vi "UnaryClientAbortTest.vi"() -> (0 "Array of Error Description":T1)   [LabVIEW 2019]
uses:
  gRPC_ATS/TestUtility/utility.llb/array of error description.ctl
  gRPC_ATS/TestUtility/utility.llb/error description.ctl
  gRPC_ATS/TestUtility/utility.llb/error type.ctl
  Generated_client/RPC Messages/helloworld_HelloReply.ctl
  Generated_client/Generated_client.lvlib
panel:
  out "Pass":bool
  in  "error in (no error)":errorcluster
  in  "Server VI path":path=path "Generated_server/Run Service.vi"
  in  "Client VI Path":path=path "Generated_client/gRPC Client Test.vi"
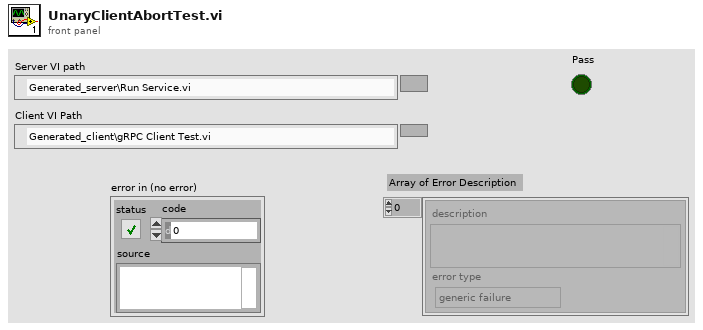
[diagram p1: front panel]
types:
  T1 = typedef "array of error description.ctl" = T2[]
  T2 = typedef "error description.ctl" = cluster{"description":string, "error type":T3}
  T3 = typedef "error type.ctl" = enum32{"generic failure", "boundary case", "precision", "expected error"}
  T4 = typedef "Generated_client.lvlib/helloworld_HelloReply.ctl" = cluster{"message":string}
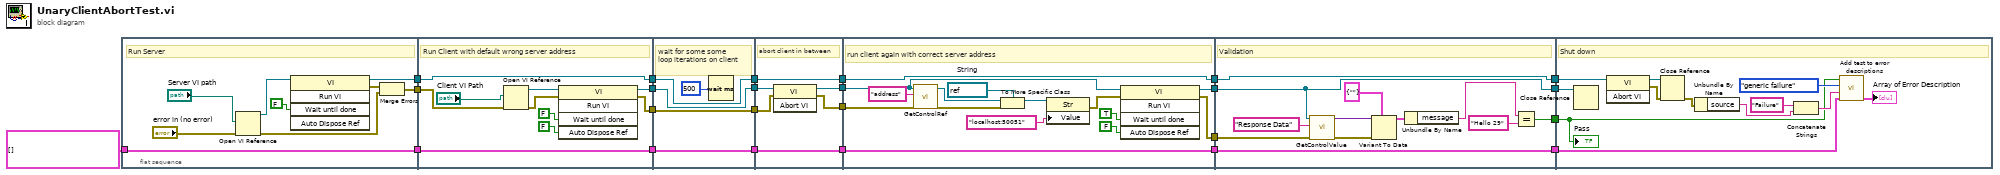
[diagram p0: block diagram]
diagram:
  n1 = flat-sequence {
    tunnel: T1 [] ("error descriptions in") -> [w29]
    tunnel: [w29] -> w23
    tunnel: [w28] -> w21
    tunnel: [w25] -> w20
    tunnel: w23 -> [w42]
    tunnel: [w42] -> w19
    tunnel: [w41] -> w17
    tunnel: w21 -> [w41]
    tunnel: w20 -> [w40]
    tunnel: [w35] -> w15
    tunnel: [w34] -> w13
    tunnel: w19 -> [w48]
    tunnel: [w48] -> w18
    tunnel: w17 -> [w47]
    tunnel: [w47] -> w16
    tunnel: w15 -> [w46]
    tunnel: [w46] -> w14
    tunnel: w13 -> [w45]
    tunnel: [w45] -> w12
    tunnel: w18 -> [w54]
    tunnel: [w54] -> w11
    tunnel: w16 -> [w53]
    tunnel: [w53] -> w9
    tunnel: w14 -> [w52]
    tunnel: [w49] -> w7
    tunnel: w12 -> [w51]
    tunnel: [w50] -> w5
    tunnel: w11 -> [w69]
    tunnel: [w69] -> w10
    tunnel: w9 -> [w68]
    tunnel: [w68] -> w8
    tunnel: w7 -> [w63]
    tunnel: [w67] -> w6
    tunnel: w5 -> [w62]
    tunnel: [w66] -> w4
    tunnel: w10 -> [w81]
    tunnel: [w81] -> w22
    tunnel: w8 -> [w80]
    tunnel: w6 -> [w77]
    tunnel: w4 -> [w75]
    tunnel: [w80] -> w3
    tunnel: [w77] -> w2
    tunnel: [w70] -> w1
    tunnel: w22 -> [w88]
    tunnel: w3 -> [w84]
    tunnel: w2 -> [w83]
    tunnel: w1 -> [w82]
    frame #0 {
      # "Run Server"
      n2 = Open VI Reference(vi path="Server VI path", error in (no error)="error in (no error)") -> (vi reference=w31:refnum<vi>, error out=w27:errorcluster)  [unwired: 4 in]
      n3 = invoke class="VI" method="Run VI"(reference=w31, "Wait until done"=FALSE ("Wait Until Done")) -> (reference out=w28:refnum<vi>, error out=w26:errorcluster)  [unwired: 3 in, 3 out]
      n4 = Merge Errors(w26, w27) -> (w25:errorcluster)
    }
    frame #1 {
      # "Run Client with default wrong server address"
      n5 = Open VI Reference(vi path="Client VI Path", error in (no error)=w40) -> (vi reference=w39:refnum<vi>, error out=w38:errorcluster)  [unwired: 4 in]
      n6 = invoke class="VI" method="Run VI"(reference=w39, error in=w38, "Wait until done"=FALSE ("Wait Until Done"), "Auto Dispose Ref"=FALSE ("Auto Dispose Reference")) -> (reference out=w35:refnum<vi>, error out=w34:errorcluster)  [unwired: 1 in, 3 out]
    }
    frame #2 {
      # "wait for some some loop iterations on client"
      n7 = Wait (ms)(milliseconds to wait=u32 500) -> ()  [unwired: 1 out]
    }
    frame #3 {
      # "abort client in between"
      n8 = invoke class="VI" method="Abort VI"(reference=w52, error in=w51) -> (reference out=w49:refnum<vi>, error out=w50:errorcluster)  [unwired: 1 in, 1 out]
    }
    frame #4 {
      w60 = refnum<vi> refnum  # String
      # "run client again with correct server address"
      n9 = call "GetControlRef.vi"("error in (no error)"=w62, "Control Label"="address", "VI Reference"=w63) -> ("error out"=w59:errorcluster, "Ctl Refnum"=w61:refnum<vi>)  [unwired: 7 in]
      n10 = To More Specific Class(target class=w60, reference=w61, error in=w59) -> (specific class reference=w58:refnum<vi>)  [unwired: 1 out]
      n11 = property class="Str"(reference=w58, "Value"="localhost:50051") -> (error out=w56:errorcluster)  [unwired: 1 in, 1 out]
      n12 = invoke class="VI" method="Run VI"(reference=w63, error in=w56, "Wait until done"=TRUE ("Wait Until Done"), "Auto Dispose Ref"=FALSE ("Auto Dispose Reference")) -> (reference out=w67:refnum<vi>, error out=w66:errorcluster)  [unwired: 1 in, 3 out]
    }
    frame #5 {
      # "Validation"
      n13 = call "GetControlValue.vi"("error in (no error)"=w75, "Control Label"="Response Data", "VI Reference"=w77) -> ("error out"=w79:errorcluster, "Value"=w78:variant)  [unwired: 7 in]
      n14 = Variant To Data(error in=w79, type=T4 {"message"=""} ("helloworld_HelloReply"), Variant=w78) -> (data=w73:T4)  [unwired: 1 out]
      n15 = Unbundle By Name(w73) -> ("message"=w72:string)
      n16 = Equal?(x=w72, y="Hello 29" ("message")) -> (x = y?=w70:bool)
    }
    frame #6 {
      # "Shut down"
      n17 = Close Reference(reference=w83) -> ()  [unwired: 1 in, 1 out]
      n18 = invoke class="VI" method="Abort VI"(reference=w84) -> (reference out=w86:refnum<vi>, error out=w87:errorcluster)  [unwired: 2 in, 1 out]
      n19 = Close Reference(reference=w86, error in (no error)=w87) -> (error out=w85:errorcluster)
      n20 = Unbundle By Name(w85) -> ("source"=w90:string)
      n21 = Concatenate Strings("Failure" ("string"), w90) -> (w91:string)
      n22 = call "Add test to error descriptions.vi"("error descriptions in"=w88, "error string"=w91, "error type"=error_type."generic failure", "pass"=w82) -> ("error description out"=→"Array of Error Description":T1)  [unwired: 3 in]
      "Pass" <- w82
    }
  }
